vi "csm_lumikki_instron_startLogging_poller.vi"() -> ()   [LabVIEW 2009]
uses:
  <vilib>/Utility/file.llb/Write To Spreadsheet File (DBL).vi
panel:
  out "FullScaleCha3":dbl
  out "FullScaleCha2":dbl
  out "FullScaleCha1":dbl
  out "path":path
  out "RootPath":string
  in  "Column Types":i32[][](array[ring])=[[0, 0, 0, 0, 0, 0, 0, 0]] items=["Feedback", "Direct Auxilary"]
  in  "Number of Columns":i32[](array[numeric])=[3]
  in  "Column Channels":i32[][](array[ring])=[[1, 2, 3, 0, 0, 0, 0, 0]] items=["Not Used", "Channel 1/Logging time", "Channel 2/Controlling command", "Channel 3/Controlling error", "Channel 4/Elapsed quarter-cycle counter", "Total accumulated quarter-cycle counter", "Elapsed segment counter", "Total accumulated segment counter", "Servovalve drive", "Block count", "Uncompensated servovalve drive", "Geometric compensation output 1", "Geometric compensation output 2", "Re-Sampling Filter 1", "Re-Sampling Filter 2", "Re-Sampling Filter 3", "Re-Sampling Filter 4", "Outer cascaded controller output", "Delta_P or acceleration compensation (Raw)", "Auxiliary input from the front of the IAC", "Waveform identifier", "Reserved", "Digital I/O and sample playback actions", "Reserved", "Motor current (EIB only)", "Motor instantaneous power (EIB only)", "Motot filtered power (EIB only)", "Motor speed (EIB only)", "Motor viscous loss (EIB only)"]
  in  "Interval/Buffer Parameters":T1={"Sample interval - ms (2)"=2.0, "Buffer Length (1000)"=1000, "No. of Buffers (0)"=0} {"Sample interval - ms (2)" min=0.2 format="%.1f"}
  out "Waveform Graph 2":dbl[][](graph)
  # "datalogger internal \npreferences:"
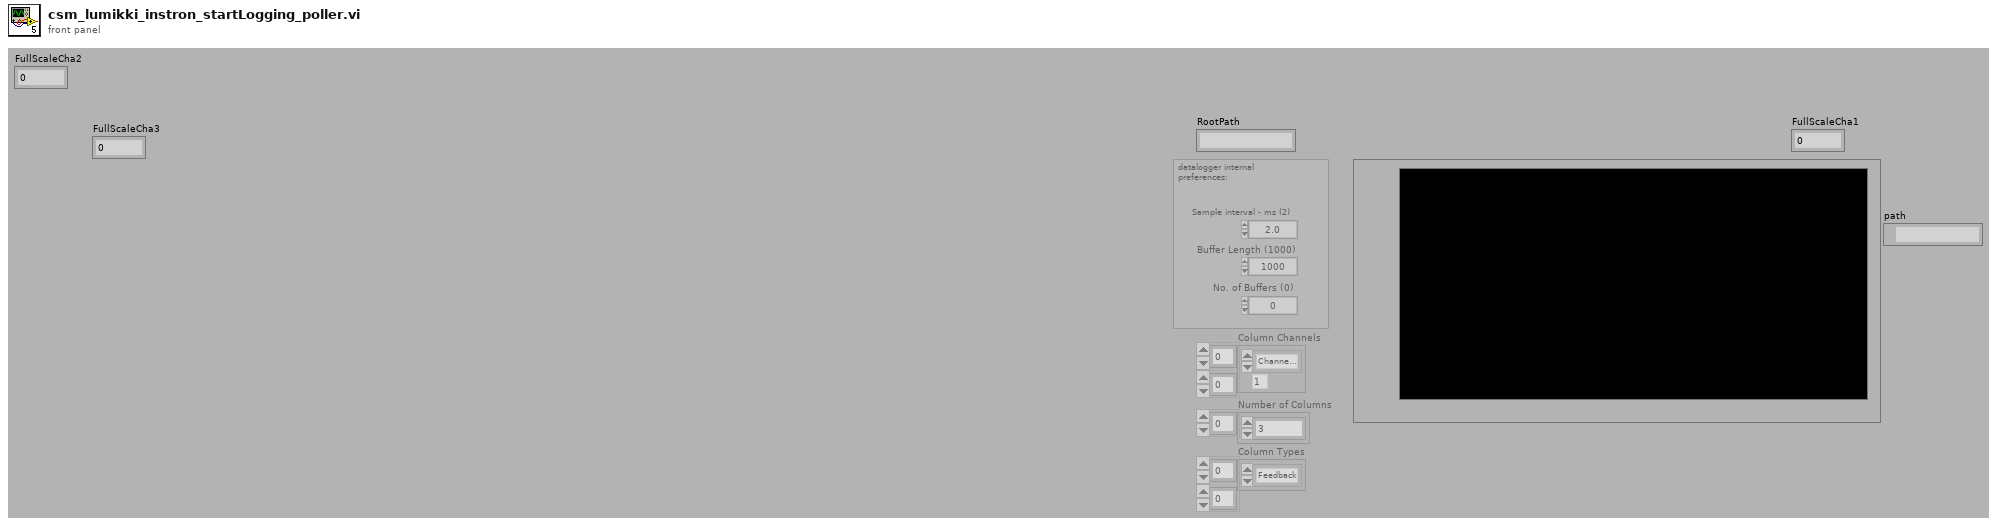
[diagram p1: front panel]
types:
  T1 = cluster{"Sample interval - ms (2)":dbl, "Buffer Length (1000)":i32, "No. of Buffers (0)":i32}
  T2 = cluster{"Name":string, "Type":i32, "SI Full Scale":dbl, "Full Scale":dbl, "Units String":string, "Display Format":string, "Gauge Length":dbl}[][]
  T3 = cluster{"Device ID":i32, "Device Name":string, "Device Type":i32}[]
  T4 = cluster{"Conversion Factors[0]":dbl, "Conversion Factors[1]":dbl, "Conversion Factors[2]":dbl, "Conversion Factors[3]":dbl, "Conversion Factors[4]":dbl, "Conversion Factors[5]":dbl, "Conversion Factors[6]":dbl, "Conversion Factors[7]":dbl, "Conversion Factors[8]":dbl}
  T5 = typedef "NI_Matrix.lvlib/RealMatrix.ctl" = dbl[][]
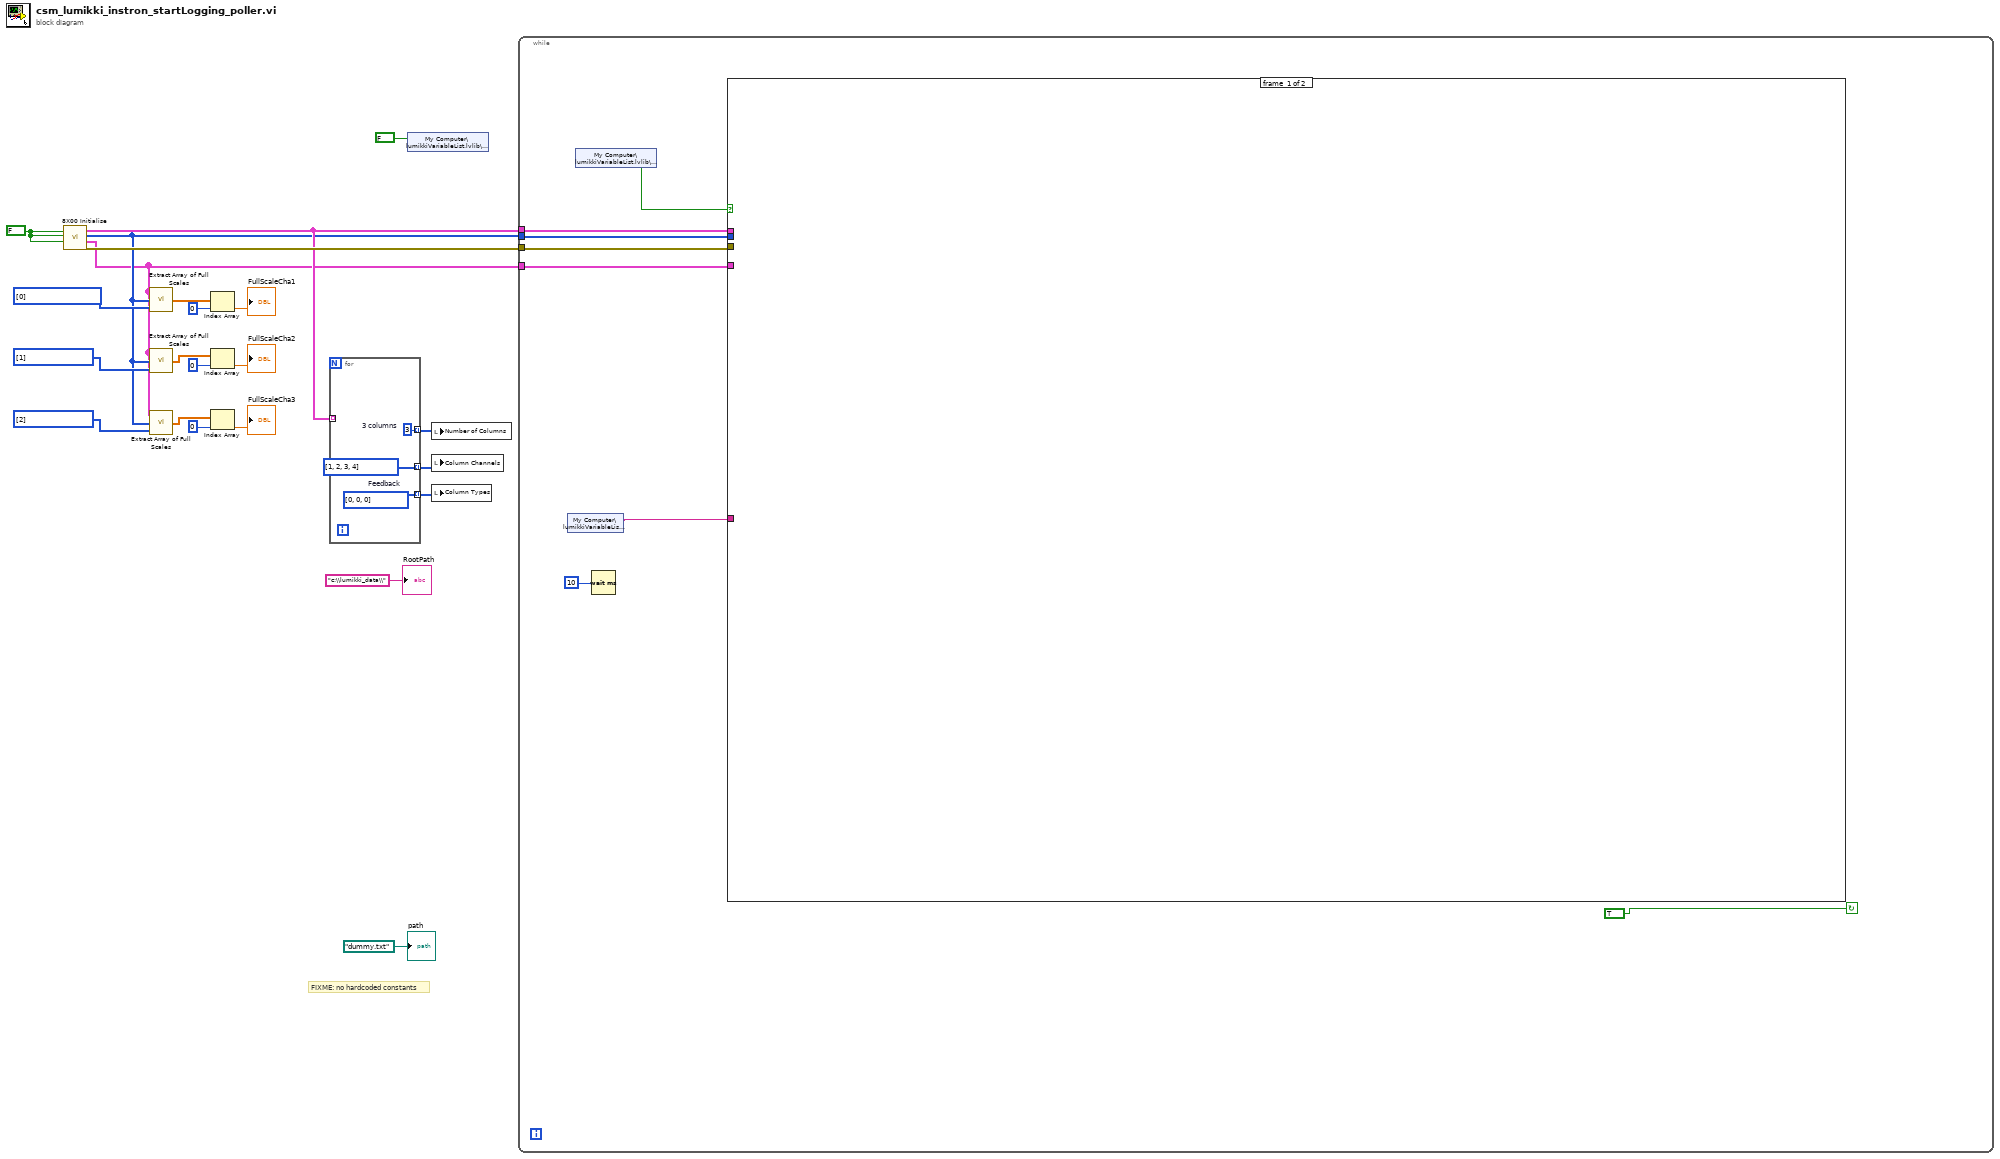
[diagram p0: block diagram]
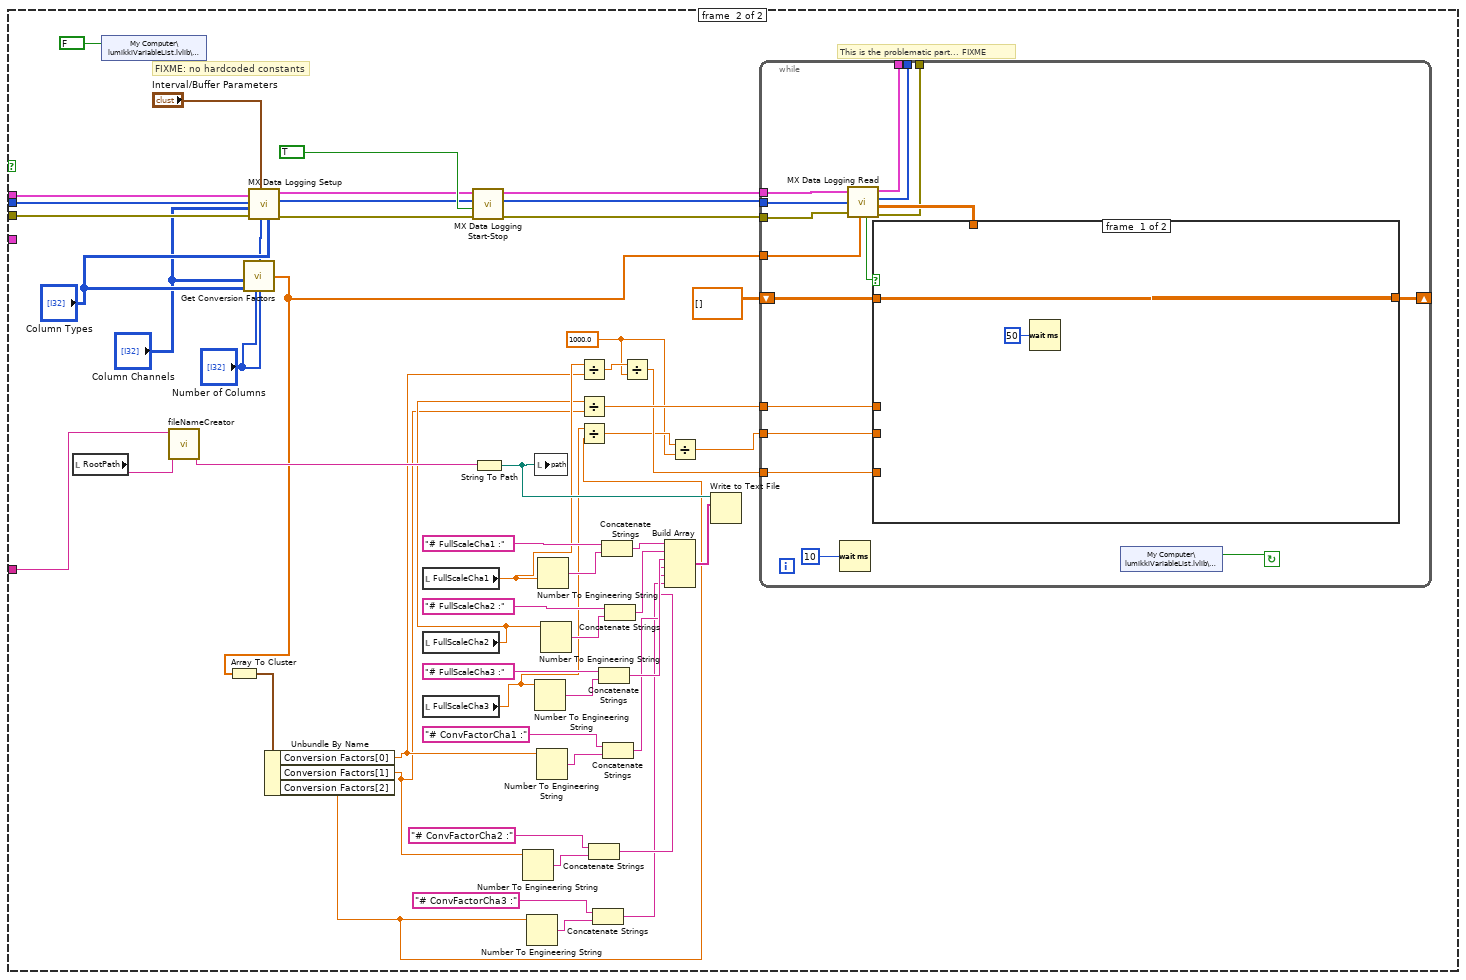
[diagram p2: hidden frame]
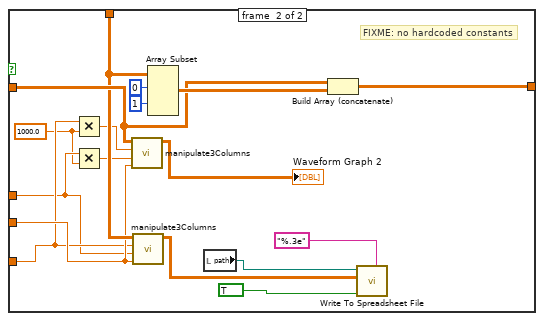
[diagram p3: hidden frame]
diagram:
  w12 = u16[] [2] items=["Channel 1", "Channel 2", "Channel 3", "Channel 4"] ("Channel")
  w13 = u16[] [1] items=["Channel 1", "Channel 2", "Channel 3", "Channel 4"] ("Channel")
  w16 = u16[] [0] items=["Channel 1", "Channel 2", "Channel 3", "Channel 4"] ("Channel")
  w23 = FALSE ("Create Console? (T)")
  # "FIXME: no hardcoded constants"
  n1 = call "8X00 Initialise.vi"("Reset?"=w23, "Create DVM? (T)"=w23, "Create Console? (T)"=w23) -> ("error out"=w22:errorcluster, "Channel Data"=w10:T2, "Axis Selector"=w11:i32[], "Axis Information"=w17:T3)  [unwired: 1 in]
  n2 = call "Extract Array of Full Scales.vi"("Channel"=w16, "Axis Selector"=w11, "Axis\nChannel"=w10) -> ("Full Scales"=w9:dbl[])
  n3 = call "Extract Array of Full Scales.vi"("Channel"=w13, "Axis Selector"=w11, "Axis\nChannel"=w10) -> ("Full Scales"=w1:dbl[])
  n4 = call "Extract Array of Full Scales.vi"("Channel"=w12, "Axis Selector"=w11, "Axis\nChannel"=w10) -> ("Full Scales"=w2:dbl[])
  n5 = Index Array(array=w9, index=0) -> (element=→"FullScaleCha1":dbl)
  n6 = Index Array(array=w1, index=0) -> (element=→"FullScaleCha2":dbl)
  n7 = Index Array(array=w2, index=0) -> (element=→"FullScaleCha3":dbl)
  n8 = for {
    tunnel: [w26] -> w20 mode=indexing
    tunnel: [w25] -> w18 mode=indexing
    tunnel: [3] -> w19 mode=indexing
    tunnel: w17 -> [_] mode=indexing
    w25 = i32[] [0, 0, 0]  # Feedback
    w26 = i32[] [1, 2, 3, 4]  # 3 columns
  }
  n9 = shared-variable "My Computer\\lumikkiVariableList.lvlib\\startLogging"(FALSE ("startLogging")) -> ()  [unwired: 1 in, 1 out]
  n10 = local write "Number of Columns"(w19) -> ()
  n11 = local write "Column Channels"(w20) -> ()
  n12 = local write "Column Types"(w18) -> ()
  n13 = while {
    tunnel: w17 -> [w32]
    tunnel: w11 -> [w31]
    tunnel: w22 -> [w30]
    tunnel: w10 -> [w27]
    stop <- TRUE continue-if-true
    n14 = shared-variable "My Computer\\lumikkiVariableList.lvlib\\expId"() -> (w28:string)  [unwired: 1 in, 1 out]
    n15 = shared-variable "My Computer\\lumikkiVariableList.lvlib\\startLogging"() -> (w29:bool)  [unwired: 1 in, 1 out]
    n16 = Wait (ms)(milliseconds to wait=u32 10) -> ()  [unwired: 1 out]
    n17 = case shown="True" w29 {
      tunnel: w32 -> [_ w78]
      tunnel: w31 -> [_ w79]
      tunnel: w30 -> [_ w80]
      tunnel: w28 -> [_ w77]
      tunnel: w27 -> [_ _]
      frame #0 {
      }
      frame #1 {
        w37 = 1000.0 ("y")
        # "FIXME: no hardcoded constants"
        # "This is the problematic part... FIXME"
        n18 = local read "RootPath"() -> (w70:string)
        n19 = shared-variable "My Computer\\lumikkiVariableList.lvlib\\startLogging"(FALSE ("startLogging")) -> ()  [unwired: 1 in, 1 out]
        n20 = call "fileNameCreator.vi"("folder"=w70, "Measurement ID"=w77) -> ("concatenated string"=w71:string)  [unwired: 9 in]
        n21 = call "Get Conversion Factors.vi"("Column Channels"="Column Channels", "Column Types"="Column Types", "Number of Columns"="Number of Columns") -> ("Conversion Factors"=w58:dbl[])  [unwired: 2 in]
        n22 = Array To Cluster(array=w58) -> (cluster=w57:T4)
        n23 = call "MX Data Logging Setup.vi"("Column Types"="Column Types", "Number of Columns"="Number of Columns", "Interval/Buffer Parameters"="Interval/Buffer Parameters", "error in (no error)"=w80, "Column Channels"="Column Channels", "Axis Selector"=w79, "Axis Information"=w78) -> ("error out"=w84:errorcluster, "Axis Selector copy"=w73:i32[], "Axis Information out"=w74:T3)  [unwired: 1 out]
        n24 = Unbundle By Name(w57) -> ("Conversion Factors[0]"=w46:dbl, "Conversion Factors[1]"=w44:dbl, "Conversion Factors[2]"=w41:dbl)
        n25 = local read "FullScaleCha1"() -> (w47:dbl)
        n26 = local read "FullScaleCha2"() -> (w45:dbl)
        n27 = local read "FullScaleCha3"() -> (w42:dbl)
        n28 = call "MX Data Logging Start-Stop.vi"("error in (no error)"=w84, "Start (T)"=TRUE, "Axis Selector"=w73, "Axis Information"=w74) -> ("error out"=w81:errorcluster, "Axis Selector copy"=w82:i32[], "Axis Information out"=w83:T3)  [unwired: 4 in]
        n29 = String To Path(string=w71) -> (path=w69:path)
        n30 = Number To Engineering String(4:w44) -> (0:w52:string)  [unwired: 3 in]
        n31 = Number To Engineering String(4:w41) -> (0:w49:string)  [unwired: 3 in]
        n32 = local write "path"(w69) -> ()
        n33 = Number To Engineering String(4:w42) -> (0:w59:string)  [unwired: 3 in]
        n34 = Number To Engineering String(4:w46) -> (0:w55:string)  [unwired: 3 in]
        n35 = Number To Engineering String(4:w47) -> (0:w65:string)  [unwired: 3 in]
        n36 = Number To Engineering String(4:w45) -> (0:w63:string)  [unwired: 3 in]
        n37 = Divide(x=w47, y=w46) -> (x/y=w40:dbl)
        n38 = Divide(x=w45, y=w44) -> (x/y=w43:dbl)
        n39 = Divide(x=w42, y=w41) -> (x/y=w38:dbl)
        n40 = Concatenate Strings("# ConvFactorCha2 :", w52) -> (w51:string)
        n41 = Concatenate Strings("# ConvFactorCha3 :", w49) -> (w48:string)
        n42 = Concatenate Strings("# FullScaleCha3 :", w59) -> (w60:string)
        n43 = Concatenate Strings("# FullScaleCha1 :", w65) -> (w67:string)
        n44 = Concatenate Strings("# ConvFactorCha1 :", w55) -> (w54:string)
        n45 = Concatenate Strings("# FullScaleCha2 :", w63) -> (w62:string)
        n46 = Divide(x=w40, y=w37) -> (x/y=w39:dbl)
        n47 = Build Array(w67, w62, w60, w54, w51, w48) -> (w68:string[])
        n48 = Divide(x=w38, y=w37) -> (x/y=w36:dbl)
        n49 = Write to Text File(file (use dialog)=w69, text=w68) -> ()  [unwired: 2 in, 3 out]
        n50 = while {
          tunnel: [w95] -> _
          tunnel: [w96] -> _
          tunnel: w81 -> [w99]
          tunnel: w58 -> [w98]
          tunnel: w82 -> [w100]
          tunnel: w83 -> [w101]
          tunnel: [w94] -> _
          shift-right: [w93] -> _
          shift-left: dbl[][] [] -> [w92]
          tunnel: w39 -> [w90]
          tunnel: w43 -> [w89]
          tunnel: w36 -> [w88]
          stop <- w91 continue-if-true
          n51 = Wait (ms)(milliseconds to wait=u32 10) -> ()  [unwired: 1 out]
          n52 = call "MX Data Logging Read.vi"("Axis Information"=w101, "Axis Selector"=w100, "error in (no error)"=w99, "Conversion Values (100)"=w98) -> ("Axis Information copy"=w94:T3, "Axis Selector copy"=w96:i32[], "Data Available"=w97:bool, "Collected Data - Eng Units"=w102:dbl[][], "error out"=w95:errorcluster)  [unwired: 2 out]
          n53 = case shown="True" w97 {
            tunnel: w102 -> [_ w113]
            tunnel: [w104 w118] -> w93
            tunnel: w92 -> [w104 w117]
            tunnel: w90 -> [_ w110]
            tunnel: w89 -> [_ w108]
            tunnel: w88 -> [_ w111]
            frame #0 {
              n54 = Wait (ms)(milliseconds to wait=u32 50) -> ()  [unwired: 1 out]
            }
            frame #1 {
              w107 = 1000.0 ("y")
              # "FIXME: no hardcoded constants"
              n55 = Multiply(x=w110, y=w107) -> (x*y=w109:dbl)
              n56 = Multiply(x=w108, y=w107) -> (x*y=w106:dbl)
              n57 = call "manipulate3Columns.vi"("Col2Mul"=w111, "Col1Mul"=w106, "Col0Mul"=w109, "Real Matrix"=w117) -> ("submatrix"=→"Waveform Graph 2":T5)  [unwired: 7 in]
              n58 = call "manipulate3Columns.vi"("Col2Mul"=w111, "Col1Mul"=w108, "Col0Mul"=w110, "Real Matrix"=w113) -> ("submatrix"=w112:T5)  [unwired: 7 in]
              n59 = Array Subset(array=w113, index (row)=0 ("index"), length (row)=1 ("length")) -> (w119:dbl[][])  [unwired: 2 in]
              n60 = local read "path"() -> (w114:path)
              n61 = Build Array (concatenate)(w117, w119) -> (w118:dbl[][])
              n62 = call-poly <vilib>:"Write To Spreadsheet File.vi"("format (%.3f)"="%.3e", "append to file? (new file:F)"=TRUE, "2D data"=w112, "file path (dialog if empty)"=w114) -> ()  [unwired: 4 in, 1 out]
            }
          }
          n63 = shared-variable "My Computer\\lumikkiVariableList.lvlib\\loggingIsOn"() -> (w91:bool)  [unwired: 1 in, 1 out]
        }
      }
    }
  }
  "RootPath" <- "c:\\lumikki_data\\" ("RootPath")
  "path" <- path "dummy.txt" ("path")
